vi "MecaDrivePoseEst2_InterpRecord_New.vi"(9 "ModulePositions":T1 {"RearRight" format="%19.3f"; "RearLeft" format="%19.3f"; "FrontRight" format="%19.3f"; "FrontLeft" format="%19.3f"}, 10 "GyroAngle":T4 {"SIN" format="%13.4f"; "COS" format="%13.4f"; "VALUE" format="%13.4f"}, 11 "M_POSE_Meters":T2 {"ROTATION"."SIN" format="%13.4f"; "ROTATION"."COS" format="%13.4f"; "ROTATION"."VALUE" format="%13.4f"; "TRANSLATION"."Y" format="%14.3f"; "TRANSLATION"."X" format="%14.3f"}) -> (3 "MECA_DRIVE_POSE_EST2_INTERP_RECORD":T5 {"ModulePositions"."RearRight" format="%19.3f"; "ModulePositions"."RearLeft" format="%19.3f"; "ModulePositions"."FrontRight" format="%19.3f"; "ModulePositions"."FrontLeft" format="%19.3f"; "GyroAngle"."SIN" format="%13.4f"; "GyroAngle"."COS" format="%13.4f"; "GyroAngle"."VALUE" format="%13.4f"; "PoseMeters"."ROTATION"."SIN" format="%13.4f"; "PoseMeters"."ROTATION"."COS" format="%13.4f"; "PoseMeters"."ROTATION"."VALUE" format="%13.4f"; "PoseMeters"."TRANSLATION"."Y" format="%14.3f"; "PoseMeters"."TRANSLATION"."X" format="%14.3f"})   [LabVIEW 2019, in "Trajectory_Library.lvlib"]
doc: "Mecal Drive Pose Estimate 2 -- Interporatable Record\n\nRepresents an odometry record. The record contains the inputs provided as well as the pose that was observed based on these inputs, as well as the previous record and its inputs.\n\nConstructs an Interpolation Record with the specified parameters.\n\nThis is an internal routine. It should NOT be used by the end user."
uses:
  Trajectory_Library.lvlib
  TypeDef/MECA_DRIVE_POSE_EST2_INTERP_RECORD.ctl
  TypeDef/POSE2D.ctl
  TypeDef/TRANSLATION2D.ctl
  TypeDef/ROTATION2D.ctl
  TypeDef/MECA_WHEEL_POSITIONS.ctl
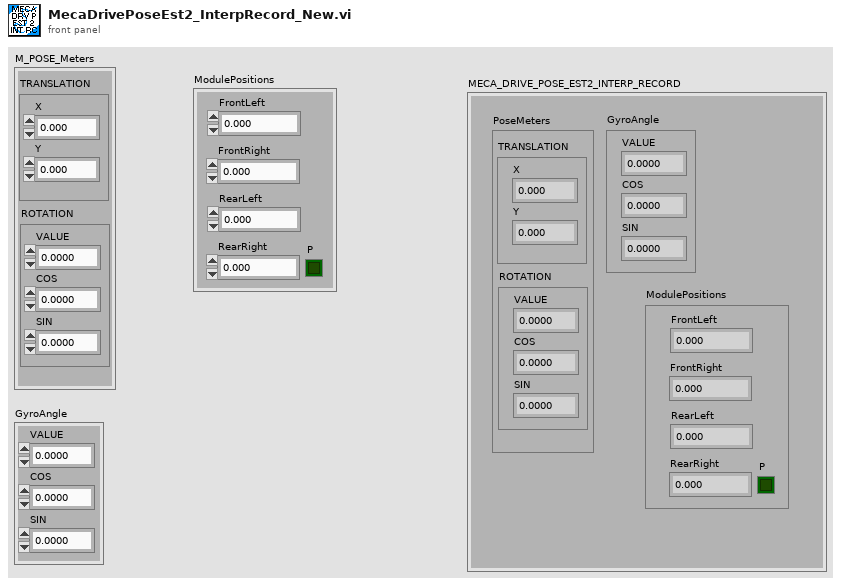
[diagram p1: front panel]
types:
  T1 = typedef "Trajectory_Library.lvlib/MECA_WHEEL_POSITIONS.ctl" = cluster{"FrontLeft":dbl, "FrontRight":dbl, "RearLeft":dbl, "RearRight":dbl, "P":bool}
  T2 = typedef "Trajectory_Library.lvlib/POSE2D.ctl" = cluster{"TRANSLATION":T3, "ROTATION":T4}
  T3 = typedef "Trajectory_Library.lvlib/TRANSLATION2D.ctl" = cluster{"X":dbl, "Y":dbl}
  T4 = typedef "Trajectory_Library.lvlib/ROTATION2D.ctl" = cluster{"VALUE":dbl, "COS":dbl, "SIN":dbl}
  T5 = typedef "Trajectory_Library.lvlib/MECA_DRIVE_POSE_EST2_INTERP_RECORD.ctl" = cluster{"PoseMeters":T2, "GyroAngle":T4, "ModulePositions":T1}
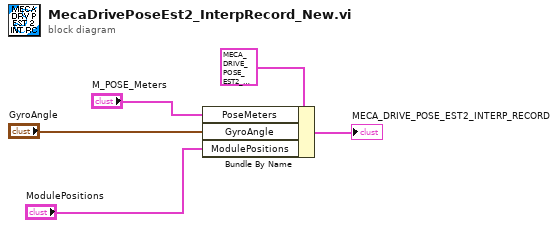
[diagram p0: block diagram]
diagram:
  n1 = Bundle By Name(cluster=T5 {"PoseMeters"={"TRANSLATION"={"X"=0.0, "Y"=0.0}, "ROTATION"={"VALUE"=0.0, "COS"=1.0, "SIN"=0.0}}, "GyroAngle"={"VALUE"=0.0, "COS"=1.0, "SIN"=0.0}, "ModulePositions"={"FrontLeft"=0.0, "FrontRight"=0.0, "RearLeft"=0.0, "RearRight"=0.0, "P"=FALSE}} ("MECA_DRIVE_POSE_EST2_INTERP_RECORD"), "PoseMeters"="M_POSE_Meters", "GyroAngle"="GyroAngle", "ModulePositions"="ModulePositions") -> (→"MECA_DRIVE_POSE_EST2_INTERP_RECORD":T5)
